vi "Forklift.vi"() -> ()   [LabVIEW 2014]
uses:
  <vilib>/Rock Robotics/WPI/RobotDrive/WPI_RobotDriveGetSetRefNum.vi
  <vilib>/Rock Robotics/WPI/Joystick/WPI_JoystickGetSetRefNum.vi
  <vilib>/Rock Robotics/Network Tables/SD Write Boolean Array.vi
  <vilib>/Rock Robotics/Network Tables/SD Write Numeric Array.vi
panel:
  in  "Y Axis - Operator":dbl
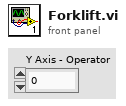
[diagram p1: front panel]
types:
  T1 = typedef "WPI_RobotDriveDevRef.ctl" = cluster{"DevStatus":errorcluster, "Motors[]":T2[], "Square Inputs":bool, "Max Output":dbl}
  T2 = typedef "WPI_MotorControlDeviceRef.ctl" = cluster{"DeviceStatus":errorcluster, "Type":T3, "PWM":cluster{"Controller":T4, "PWM Channel":T5, "DeadBand":T6}, "CAN":cluster{"Device Number":u8, "Control Mode":T7, "Semaphore":T8, "Max Vout":dbl, "TalonSRX Control Mode":T9}, "Invert":bool, "TransformRef":T10, "InvTransformRef":T10}
  T3 = typedef "WPI_MotorControlType.ctl" = enum16{"PWM", "CAN", "CANTalonSRX"}
  T4 = typedef "FPGA_TypedefDigitalModule.ctl" = enum16{"Controller 1"}
  T5 = typedef "FPGA_DIOPWMChannel.ctl" = enum8{"PWM 0", "PWM 1", "PWM 2", "PWM 3", "PWM 4", "PWM 5", "PWM 6", "PWM 7", "PWM 8", "PWM 9", "PWM MXP 0", "PWM MXP 1", "PWM MXP 2", "PWM MXP 3", "PWM MXP 4", "PWM MXP 5", "PWM MXP 6", "PWM MXP 7", "PWM MXP 8", "PWM MXP 9", "Invalid"}
  T6 = typedef "WPI_PWMDeadband.ctl" = cluster{"Name":string, "maxPositivePwm":i32, "minPositivePwm":i32, "centerPwm":i32, "maxNegativePwm":i32, "minNegativePwm":i32, "angularRange":u16}
  T7 = typedef "WPI_CANJaguar_ControlMode.ctl" = enum8{"Percent VBus", "Current", "Speed", "Position", "Voltage"}
  T8 = typedef "Semaphore RefNum" = refnum<k1>
  T9 = typedef "WPI_CANTalonSRX_APIControlMode.ctl" = enum8{"Percent VBus", "Speed", "Position", "Slave", "Unchanged / Invalid"}
  T10 = typedef "WPI_PWMTransform_ConPane.ctl" = refnum<vi>
  T11 = typedef "WPI_JoystickDevRef.ctl" = cluster{"Device":T12}
  T12 = typedef "WPI_JoystickDeviceEnum.ctl" = enum16{"USB 0", "USB 1", "USB 2", "USB 3", "USB 4", "USB 5"}
  T13 = cluster{"Buttons[0]":bool, "Buttons[1]":bool, "Buttons[2]":bool, "Buttons[3]":bool, "Buttons[4]":bool, "Buttons[5]":bool, "Buttons[6]":bool, "Buttons[7]":bool, "Buttons[8]":bool}
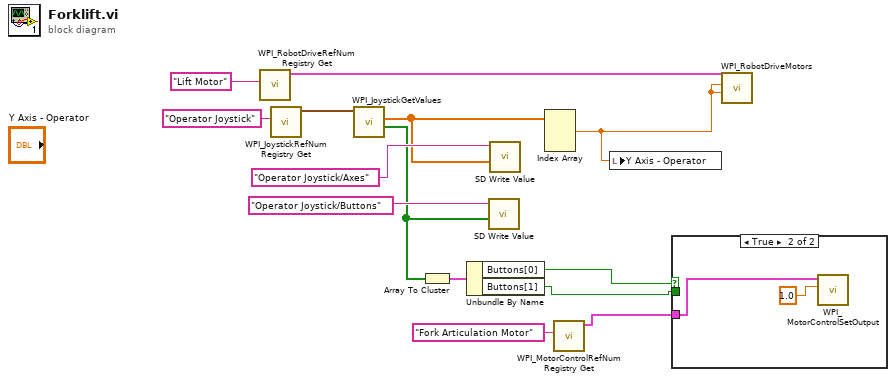
[diagram p0: block diagram]
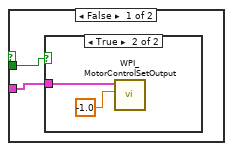
[diagram p2: hidden frame]
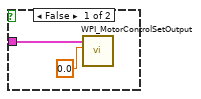
[diagram p3: hidden frame]
diagram:
  n1 = call <vilib>:"WPI_RobotDriveRefNum Registry Get.vi"("refnum name"="Lift Motor") -> ("RobotDriveDevRef"=w8:T1)  [unwired: 9 in, 1 out]
  n2 = call <vilib>:"WPI_JoystickRefNum Registry Get.vi"("refnum name"="Operator Joystick") -> ("JoystickDevRef"=w11:T11)  [unwired: 9 in, 1 out]
  n3 = call <vilib>:"WPI_JoystickGetValues.vi"("JoystickDevRef"=w11) -> ("Buttons"=w5:bool[], "Axes"=w9:dbl[])  [unwired: 6 in, 3 out]
  n4 = Array To Cluster(array=w5) -> (cluster=w4:T13)
  n5 = Unbundle By Name(w4) -> ("Buttons[0]"=w1:bool, "Buttons[1]"=w2:bool)
  n6 = call-poly <vilib>:"SD Write Value.vi"("Boolean Array"=w5, "Name"="Operator Joystick/Buttons") -> ()  [unwired: 8 in, 2 out]
  n7 = call-poly <vilib>:"SD Write Value.vi"("Numeric Array"=w9, "Name"="Operator Joystick/Axes") -> ()  [unwired: 8 in, 2 out]
  n8 = Index Array "Index Array"(array=w9) -> (element #1=w6:dbl)  [unwired: 3 in, 2 out]
  n9 = call <vilib>:"WPI_MotorControlRefNum Registry Get.vi"("refnum name"="Fork Articulation Motor") -> ("MotorControlDevRef"=w3:T2)  [unwired: 9 in, 1 out]
  n10 = local write "Y Axis - Operator"(w6) -> ()
  n11 = case shown="True" w1 {
    tunnel: w3 -> [w15 w22]
    tunnel: w2 -> [w16 _]
    frame False {
      n12 = case shown="True" w16 {
        tunnel: w15 -> [w18 w20]
        frame False {
          n13 = call <vilib>:"WPI_MotorControlSetOutput.vi"("Output"=0.0, "MotorControlDevRef"=w18) -> ()  [unwired: 7 in, 3 out]
        }
        frame True {
          n14 = call <vilib>:"WPI_MotorControlSetOutput.vi"("Output"=-1.0, "MotorControlDevRef"=w20) -> ()  [unwired: 7 in, 3 out]
        }
      }
    }
    frame True {
      n15 = call <vilib>:"WPI_MotorControlSetOutput.vi"("Output"=1.0, "MotorControlDevRef"=w22) -> ()  [unwired: 7 in, 3 out]
    }
  }
  n16 = call <vilib>:"WPI_RobotDriveMotors.vi"("RightSpeed"=w6, "LeftSpeed"=w6, "RobotDriveDevRef"=w8) -> ()  [unwired: 6 in, 3 out]
